vi "_FPGA_U32equal1.vi"(10 "Numeric":u32) -> (2 "=1?":bool)   [LabVIEW 2018]
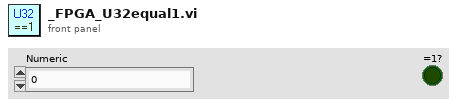
[diagram p1: front panel]
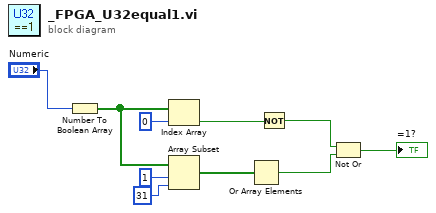
[diagram p0: block diagram]
diagram:
  n1 = Number To Boolean Array(number="Numeric") -> (Boolean array=w7:bool[])
  n2 = Index Array(array=w7, index=0) -> (element=w5:bool)
  n3 = Array Subset(array=w7, index=1, length=31) -> (w4:bool[])
  n4 = Or Array Elements(Boolean array=w4) -> (logical OR=w2:bool)
  n5 = Not(x=w5) -> (.not. x?=w3:bool)
  n6 = Not Or(1:w2, 2:w3) -> (0:→"=1?":bool)
